vi "Enqueue.vi"(7 "EnqueType (Enque)":enum16{"LossyEnque", "EnqueAtFront", "Enque"}(ring), 8 "error in (no error)":errorcluster, 9 "Message Data":variant, 10 "Message":string, 11 "MessageQueue":refnum<queue>) -> (0 "error out":errorcluster, 3 "MessageQueue":refnum<queue>)   [LabVIEW 2018, in "AcPwrModule.lvlib"]
uses:
  AcPwrModule.lvlib
  PublicAPI/Arguments/Messages/clMessage.ctl
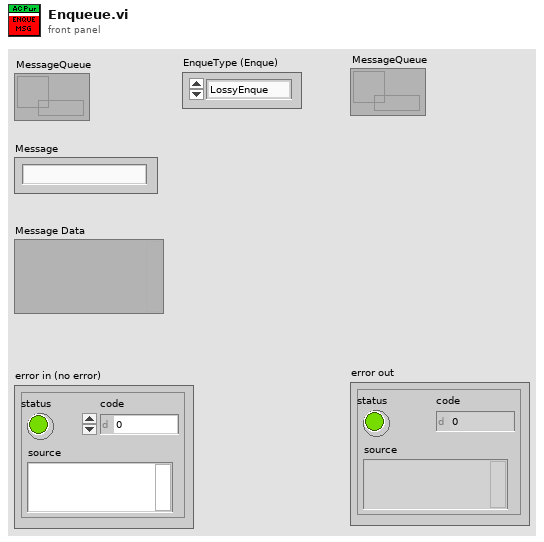
[diagram p1: front panel]
types:
  T1 = typedef "AcPwrModule.lvlib/clMessage.ctl" = cluster{"Message":string, "Message Data":variant}
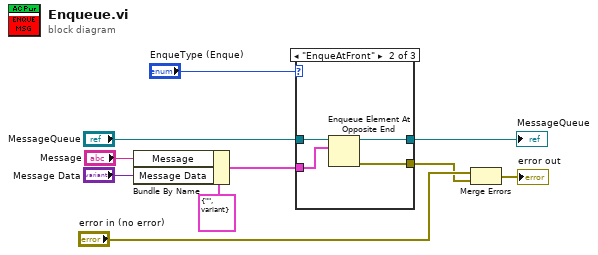
[diagram p0: block diagram]
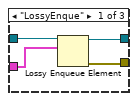
[diagram p2: hidden frame]
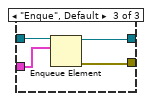
[diagram p3: hidden frame]
diagram:
  n1 = Bundle By Name(cluster=T1 {"Message"="", "Message Data"=variant} ("clMessage"), "Message"="Message", "Message Data"="Message Data") -> (w9:T1)
  n2 = case shown="\"EnqueAtFront\"" "EnqueType (Enque)" {
    tunnel: w9 -> [w11 w18 w21]
    tunnel: "MessageQueue" -> [w12 w17 w22]
    tunnel: [w13 w16 w19] -> w5
    tunnel: [w14 w15 w20] -> w3
    frame "LossyEnque" {
      n3 = Lossy Enqueue Element(queue=w12, element=w11) -> (queue out=w13:refnum<queue>, error out=w14:errorcluster)  [unwired: 1 in, 2 out]
    }
    frame "EnqueAtFront" {
      n4 = Enqueue Element At Opposite End(queue=w17, element=w18) -> (queue out=w16:refnum<queue>, error out=w15:errorcluster)  [unwired: 2 in, 1 out]
    }
    frame "Enque", Default {
      n5 = Enqueue Element(queue=w22, element=w21) -> (queue out=w19:refnum<queue>, error out=w20:errorcluster)  [unwired: 2 in, 1 out]
    }
  }
  "MessageQueue" <- w5
  n6 = Merge Errors("error in (no error)", w3) -> (→"error out":errorcluster)
